vi "Charger_Update Searching Message.vi"(5 "Status Refnum":T1, 6 "error in":errorcluster) -> (0 "error out":errorcluster)   [LabVIEW 2020]
doc: "This function updates the Status cluster status field with a search message in the following format:\n\n\"Searching for IPG in position x (1 to 6) with MICS channel x.\""
uses:
  Charger_Status Refnum.ctl
  Drivers/Charger Test Set/Charger_Input Control.ctl
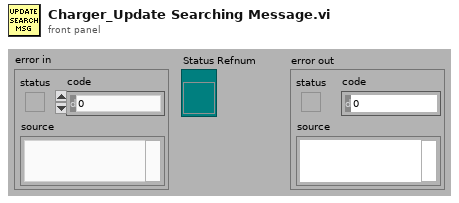
[diagram p1: front panel]
types:
  T1 = typedef "Charger_Status Refnum.ctl" = refnum<vi>
  T2 = typedef "Charger_Input Control.ctl" = cluster{"address":refnum<visa-resource-name>, "position":i32, "setpoint":dbl}
  T3 = cluster{"MICS ID":u32, "VBAT":dbl, "ChargingState":string, "VBAT Slide":dbl, "Status":string, "TemperatureLevel":dbl, "IPG_ReceivedLevel":dbl, "VBAT Target":dbl, "Charger Setpoint":dbl, "Index":i32, "Ready":bool, "Charger Inputs":T2, "MICS Inputs":cluster{"address":refnum<visa-resource-name>, "chan":u16, "ID":u32}}
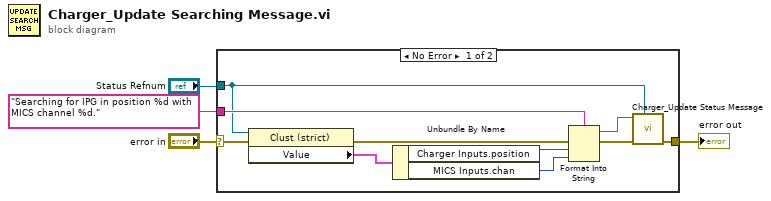
[diagram p0: block diagram]
diagram:
  n1 = case shown="No Error" "error in" {
    selector: "error in" -> [w13 w15]
    tunnel: "Status Refnum" -> [w5 _]
    tunnel: "Searching for IPG in position %d with MICS channel %d." ("Message") -> [w14 _]
    tunnel: [w7 w15] -> w1
    frame No Error {
      n2 = property class="Clust (strict)"(reference=w5, error in=w13) -> (error out=w12:errorcluster, "Value"=w11:T3)  [unwired: 1 out]
      n3 = Unbundle By Name(w11) -> ("Charger Inputs.position"=w10:i32, "MICS Inputs.chan"=w9:u16)
      n4 = Format Into String(format string=w14, error in=w12, w10, w9) -> (resulting string=w6:string, error out=w8:errorcluster)  [unwired: 1 in]
      n5 = call "Charger_Update Status Message.vi"("Status Refnum"=w5, "error in"=w8, "status message"=w6) -> ("error out"=w7:errorcluster)  [unwired: 6 in]
    }
    frame Error {
    }
  }
  "error out" <- w1
